vi "Test_ParseResultsFromAnswer.vi"   [LabVIEW 2023]
uses:
  <vilib>/addons/_JKI Toolkits/Caraya/classes/Assert/Assert Not Error.vi
  <vilib>/addons/_JKI Toolkits/Caraya/classes/Assert/Assert Equal Value_Variant.vi
  Classes/Communicator/Communicator.lvclass
  <vilib>/addons/_JKI Toolkits/Caraya/classes/Test/Test.lvclass
  <vilib>/addons/_JKI Toolkits/Caraya/classes/Assert/Assert.lvclass
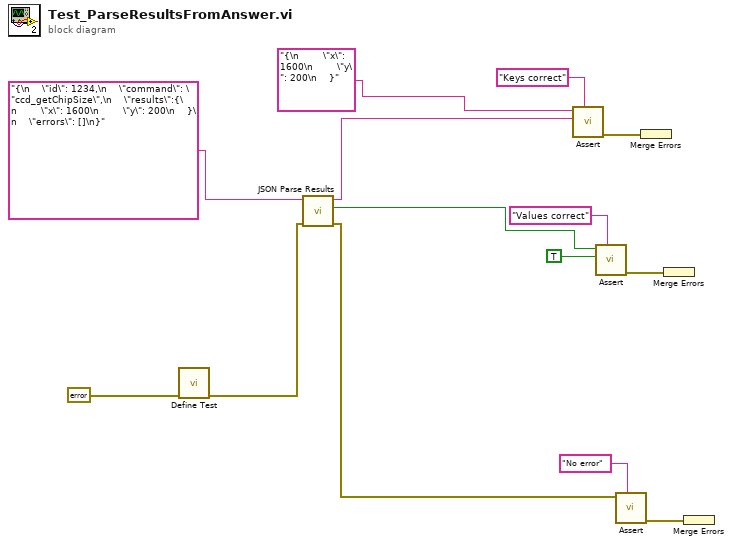
[diagram p0: block diagram]
diagram:
  n1 = call <vilib>:"Define Test.vi"("error in (no error)"=errorcluster {"status"=FALSE, "code"=0, "source"=""}) -> ("error out"=w8:errorcluster)  [unwired: 9 in, 1 out]
  n2 = call "JSON Parse Results.vi"("error in (no error)"=w8, "JSON"="{\n    \"id\": 1234,\n    \"command\": \"ccd_getChipSize\",\n    \"results\":{\n        \"x\": 1600\n        \"y\": 200\n    }\n    \"errors\": []\n}") -> ("error out"=w3:errorcluster, "key found?"=w6:bool, "results-JSON"=w7:string)  [unwired: 7 in]
  n3 = call-poly <vilib>:"Assert.vi"("Label"="Keys correct" ("Label (VI Title)"), "Y"=w7, "X"="{\n        \"x\": 1600\n        \"y\": 200\n    }") -> ("error out"=w9:errorcluster)  [unwired: 7 in, 1 out]
  n4 = call-poly <vilib>:"Assert.vi"("Label"="Values correct" ("Label (VI Title)"), "Y"=TRUE, "X"=w6) -> ("error out"=w11:errorcluster)  [unwired: 7 in, 1 out]
  n5 = call-poly <vilib>:"Assert.vi"("Label"="No error" ("Label (VI Title)"), "Not Error?"=w3) -> ("error out"=w4:errorcluster)  [unwired: 8 in, 1 out]
  n6 = Merge Errors(w9) -> ()  [unwired: 1 out]
  n7 = Merge Errors(w11) -> ()  [unwired: 1 out]
  n8 = Merge Errors(w4) -> ()  [unwired: 1 out]
